vi "RedEdge Status.vi"(8 "Error In":errorcluster) -> (0 "Error Out":errorcluster, 3 "Red Edge Status Out":T1)   [LabVIEW 2014]
uses:
  Controls/RedEdge Status.ctl
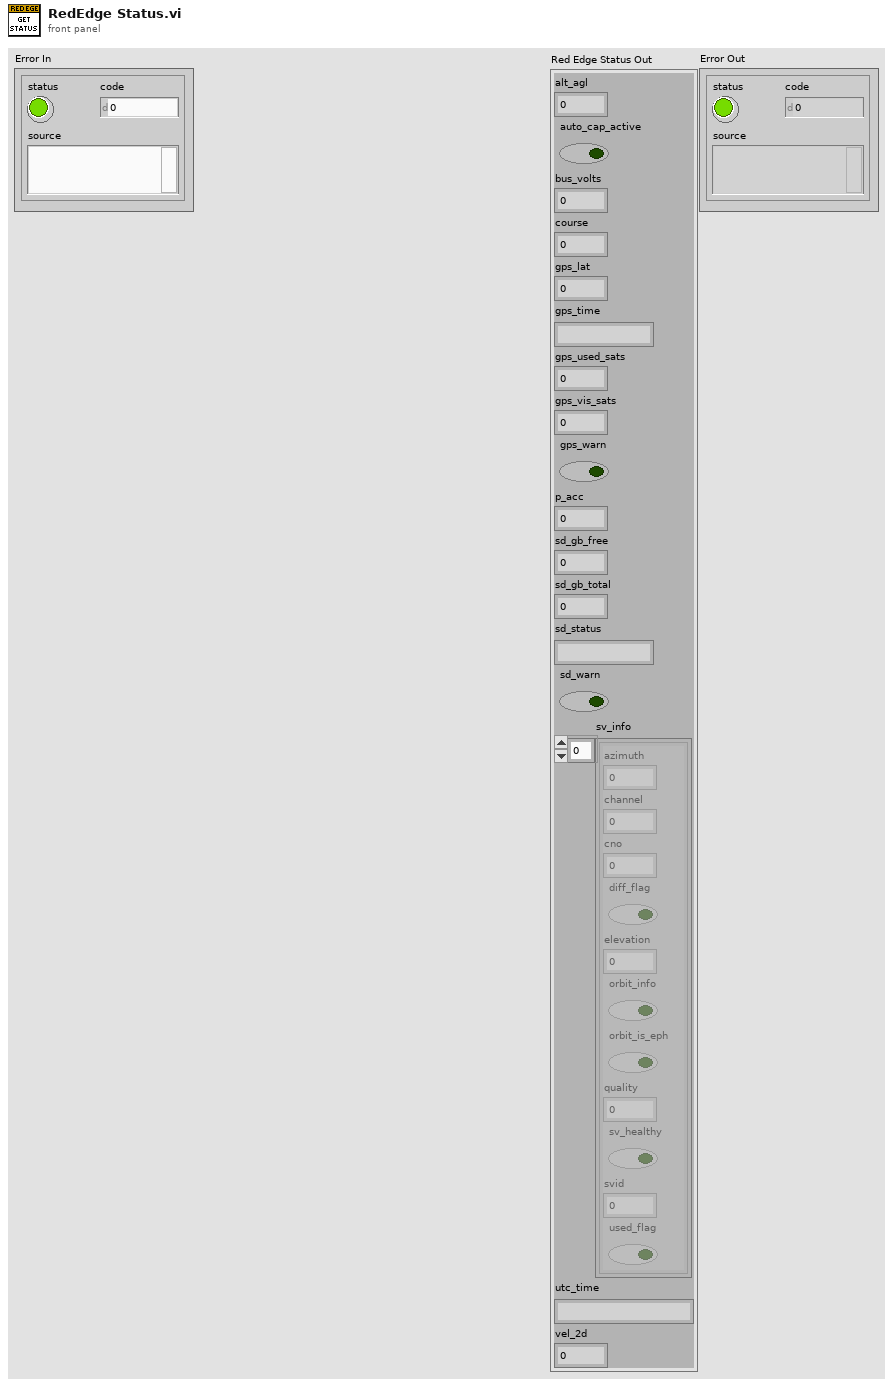
[diagram p1: front panel]
types:
  T1 = typedef "RedEdge Status.ctl" = cluster{"alt_agl":dbl, "auto_cap_active":bool, "bus_volts":i32, "course":i32, "gps_lat":dbl, "gps_time":string, "gps_used_sats":i32, "gps_vis_sats":i32, "gps_warn":bool, "p_acc":i32, "sd_gb_free":i32, "sd_gb_total":i32, "sd_status":string, "sd_warn":bool, "sv_info":cluster{"azimuth":i32, "channel":i32, "cno":i32, "diff_flag":bool, "elevation":i32, "orbit_info":bool, "orbit_is_eph":bool, "quality":i32, "sv_healthy":bool, "svid":i32, "used_flag":bool}[], "utc_time":string, "vel_2d":i32}
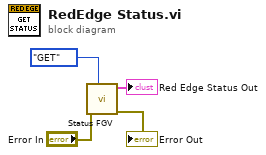
[diagram p0: block diagram]
diagram:
  n1 = call "Status FGV.vi"("Operation"=enum16{"GET", "SET"}."GET", "Error In"="Error In") -> ("Error Out"=→"Error Out":errorcluster, "Red Edge Status Out"=→"Red Edge Status Out":T1)  [unwired: 8 in]
